vi "write_attributes.vi"(8 "error in (no error)":errorcluster, 10 "attributes":T1, 11 "RidgeClassifier in":refnum<class "RidgeClassifier.lvclass">) -> (0 "error out":errorcluster, 3 "RidgeClassifier out":refnum<class "RidgeClassifier.lvclass">)   [LabVIEW 2020, in "RidgeClassifier.lvclass"]
uses:
  RidgeClassifier.lvclass
  Controls/ridge_classifier_attributes.ctl
  RidgeClassifier.lvclass/RidgeClassifier.ctl
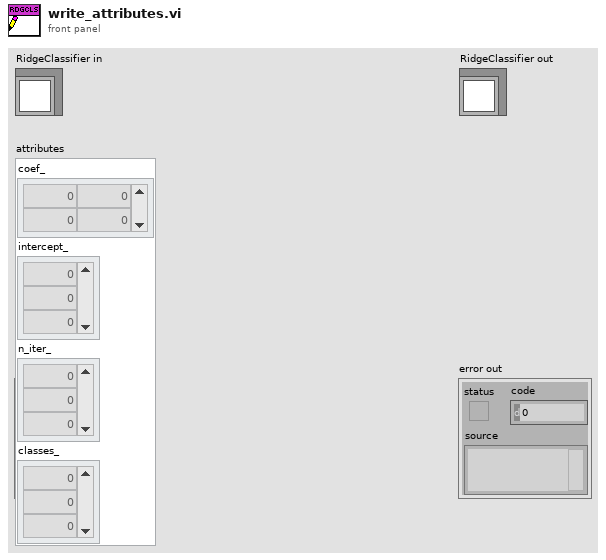
[diagram p1: front panel]
types:
  T1 = typedef "ridge_classifier_attributes.ctl" = cluster{"coef_":dbl[][], "intercept_":dbl[], "n_iter_":dbl[], "classes_":dbl[]}
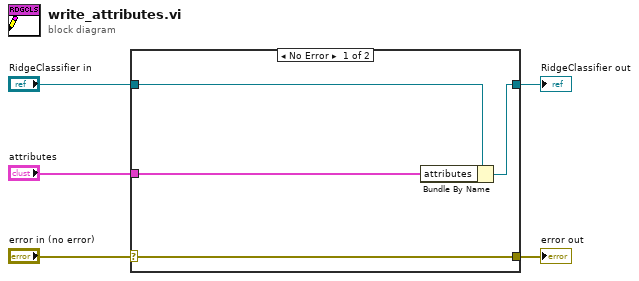
[diagram p0: block diagram]
diagram:
  n1 = case shown="No Error" "error in (no error)" {
    selector: "error in (no error)" -> [w9 w10]
    tunnel: [w9 w10] -> w4
    tunnel: [w7 w11] -> w2
    tunnel: "RidgeClassifier in" -> [w8 w11]
    tunnel: "attributes" -> [w6 _]
    frame No Error {
      n2 = Bundle By Name(cluster=w8, "attributes"=w6) -> (w7:refnum<class "RidgeClassifier.lvclass">)
    }
    frame Error {
    }
  }
  "error out" <- w4
  "RidgeClassifier out" <- w2
